vi "TBM.Init.vi"(5 "Dim Transparency":u8=99, 7 "DimRegion":enum16{"VI", "Control", "Screen"}(ring), 8 "error in (no error)":errorcluster, 9 "Position":T1, 10 "Menu Vi Reference":refnum<vi>, 11 "Control in":refnum<vi>) -> (0 "error out":errorcluster, 1 "Dimmer reference":refnum<vi>, 2 "Menu VI Refnum out":refnum<vi>, 3 "Event Registration Refnum":refnum<event-registration>)   [LabVIEW 2013, in "ToolbarMenu.lvlib"]
uses:
  ToolbarMenu.lvlib
  MenuPosition.ctl
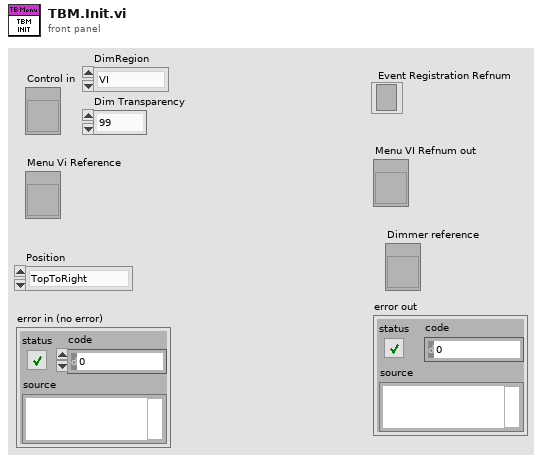
[diagram p1: front panel]
types:
  T1 = typedef "ToolbarMenu.lvlib/MenuPosition.ctl" = enum16{"TopToRight", "BottomToRight", "TopToLeft", "BottomToLeft"}
  T2 = enum32{"Invalid", "Standard", "Closed", "Hidden", "Minimized", "Maximized"}
  T3 = enum32{"Invalid", "Default", "Floating", "Floating/Auto-Hide", "Modal"}
  T4 = typedef "LVRectTypeDef.ctl" = cluster{"Left":i16, "Top":i16, "Right":i16, "Bottom":i16}
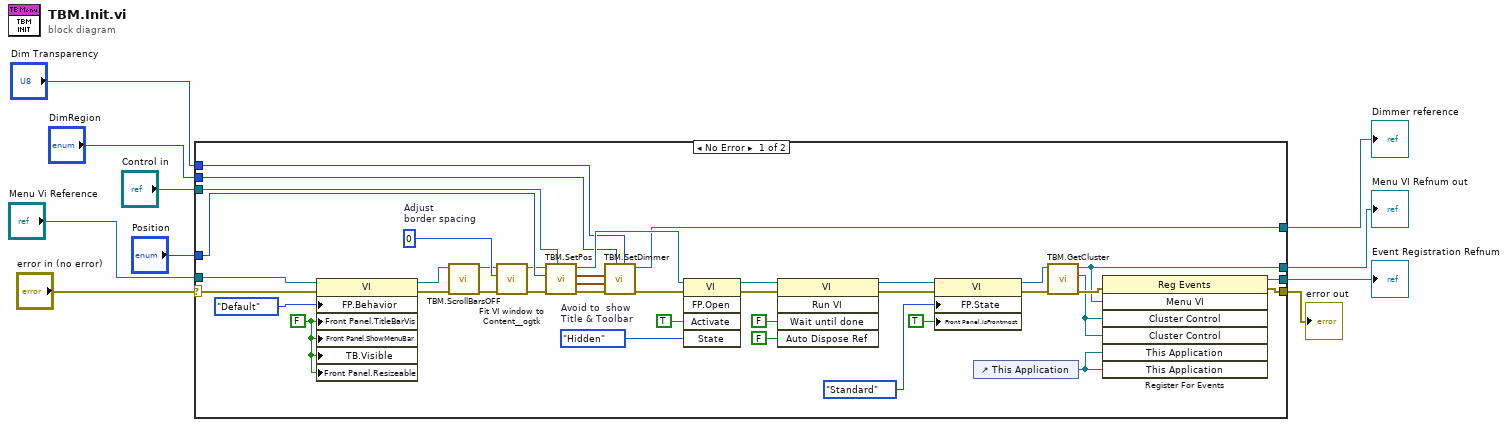
[diagram p0: block diagram]
diagram:
  n1 = case shown="No Error" "error in (no error)" {
    selector: "error in (no error)" -> [w16 w51]
    tunnel: "Position" -> [w49 _]
    tunnel: "Menu Vi Reference" -> [w17 w50]
    tunnel: "Control in" -> [w42 _]
    tunnel: [w22 w50] -> w8
    tunnel: [w30 w51] -> w7
    tunnel: [w41 _] -> w1
    tunnel: "DimRegion" -> [w27 _]
    tunnel: "Dim Transparency" -> [w26 _]
    tunnel: [w23 _] -> w2
    frame No Error {
      w40 = 0  # Adjust border spacing
      w47 = T2."Hidden"  # Avoid to  show  Title & Toolbar
      w39 = FALSE ("Front Panel Window:Title Bar Visible")
      n2 = property class="VI"(reference=w17, error in=w16, "FP.Behavior"=T3."Default" ("Front Panel Window:Behavior"), "Front Panel.TitleBarVis"=w39, "Front Panel.ShowMenuBar"=w39, "TB.Visible"=w39, "Front Panel.Resizeable"=w39) -> (reference out=w14:refnum<vi>, error out=w12:errorcluster)
      n3 = call "TBM.ScrollBarsOFF.vi"("error in (no error)"=w12, "VI in"=w14) -> ("error out"=w11:errorcluster, "VI out"=w13:refnum<vi>)  [unwired: 8 in]
      n4 = call <userlib>:"Fit VI window to Content__ogtk.vi"("error in (no error)"=w11, "border spacing (2 px)"=w40, "VI Ref (calling VI)"=w13) -> ("error out"=w20:errorcluster, "dup VI Ref"=w18:refnum<vi>)  [unwired: 3 in]
      n5 = call "TBM.SetPos.vi"("Caller Control Refnum"=w42, "error in (no error)"=w20, "Position"=w49, "Menu VI"=w18) -> ("error out"=w25:errorcluster, "Ctrl Screen Bounds"=w28:T4, "FP Screen Bounds"=w29:T4, "Menu VI"=w32:refnum<vi>)  [unwired: 4 in]
      n6 = call "TBM.SetDimmer.vi"("Dim Transparency"=w26, "DimRegion"=w27, "error in (no error)"=w25, "Ctrl Screen Bounds"=w28, "FP Screen Bounds"=w29) -> ("error out"=w24:errorcluster, "Dimmer VI out"=w23:refnum<vi>)  [unwired: 5 in]
      n7 = invoke class="VI" method="FP.Open"(reference=w32, error in=w24, "Activate"=TRUE ("Activate?"), "State"=w47) -> (reference out=w36:refnum<vi>, error out=w37:errorcluster)  [unwired: 1 in, 3 out]
      n8 = invoke class="VI" method="Run VI"(reference=w36, error in=w37, "Wait until done"=FALSE ("Wait Until Done"), "Auto Dispose Ref"=FALSE ("Auto Dispose Reference")) -> (reference out=w19:refnum<vi>, error out=w15:errorcluster)  [unwired: 1 in, 3 out]
      n9 = property class="VI"(reference=w19, error in=w15, "FP.State"=T2."Standard" ("Front Panel Window:State"), "Front Panel.IsFrontmost"=TRUE ("Activate?")) -> (reference out=w34:refnum<vi>, error out=w35:errorcluster)
      n10 = control-ref of="This Application"() -> (w38:refnum<vi>)
      n11 = call "TBM.GetCluster.vi"("error in (no error)"=w35, "Menu VI"=w34) -> ("error out"=w33:errorcluster, "Cluster Control"=w21:refnum<vi>, "Menu VI"=w22:refnum<vi>)  [unwired: 7 in]
      n12 = register-events(error in=w33, w22, w21, w21, w38, w38) -> (reference out=w41:refnum<event-registration>, error out=w30:errorcluster)  [unwired: 1 in]
    }
    frame Error {
    }
  }
  "Menu VI Refnum out" <- w8
  "error out" <- w7
  "Dimmer reference" <- w2
  "Event Registration Refnum" <- w1
